vi "GetWheaterData.vi"(11 "Locaion":string="newyork") -> (3 "WeatherString":string)   [LabVIEW 2015]
uses:
  TypeDefs/OpenWeatherMapAPI.Responce.ctl
  <vilib>/httpClient/LabVIEWHTTPClient.lvlib
panel:
  out "error out":errorcluster
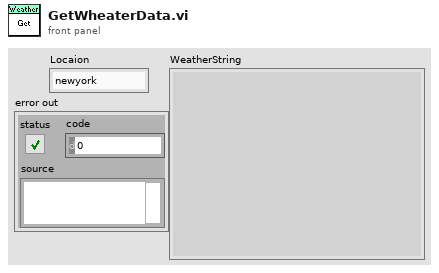
[diagram p1: front panel]
types:
  T1 = typedef "OpenWeatherMapAPI.Responce.ctl" = cluster{"weather":cluster{"main":string, "description":string}[], "main":cluster{"temp":dbl, "pressure":i32, "humidity":i32}, "wind":cluster{"speed":sgl}, "clouds":cluster{"all":i32}, "dt":u64, "sys":cluster{"country":string, "sunrise":u64, "sunset":u64}, "id":i32, "name":string, "cod":i32}
  T2 = cluster{"weather[0]":cluster{"main":string, "description":string}}
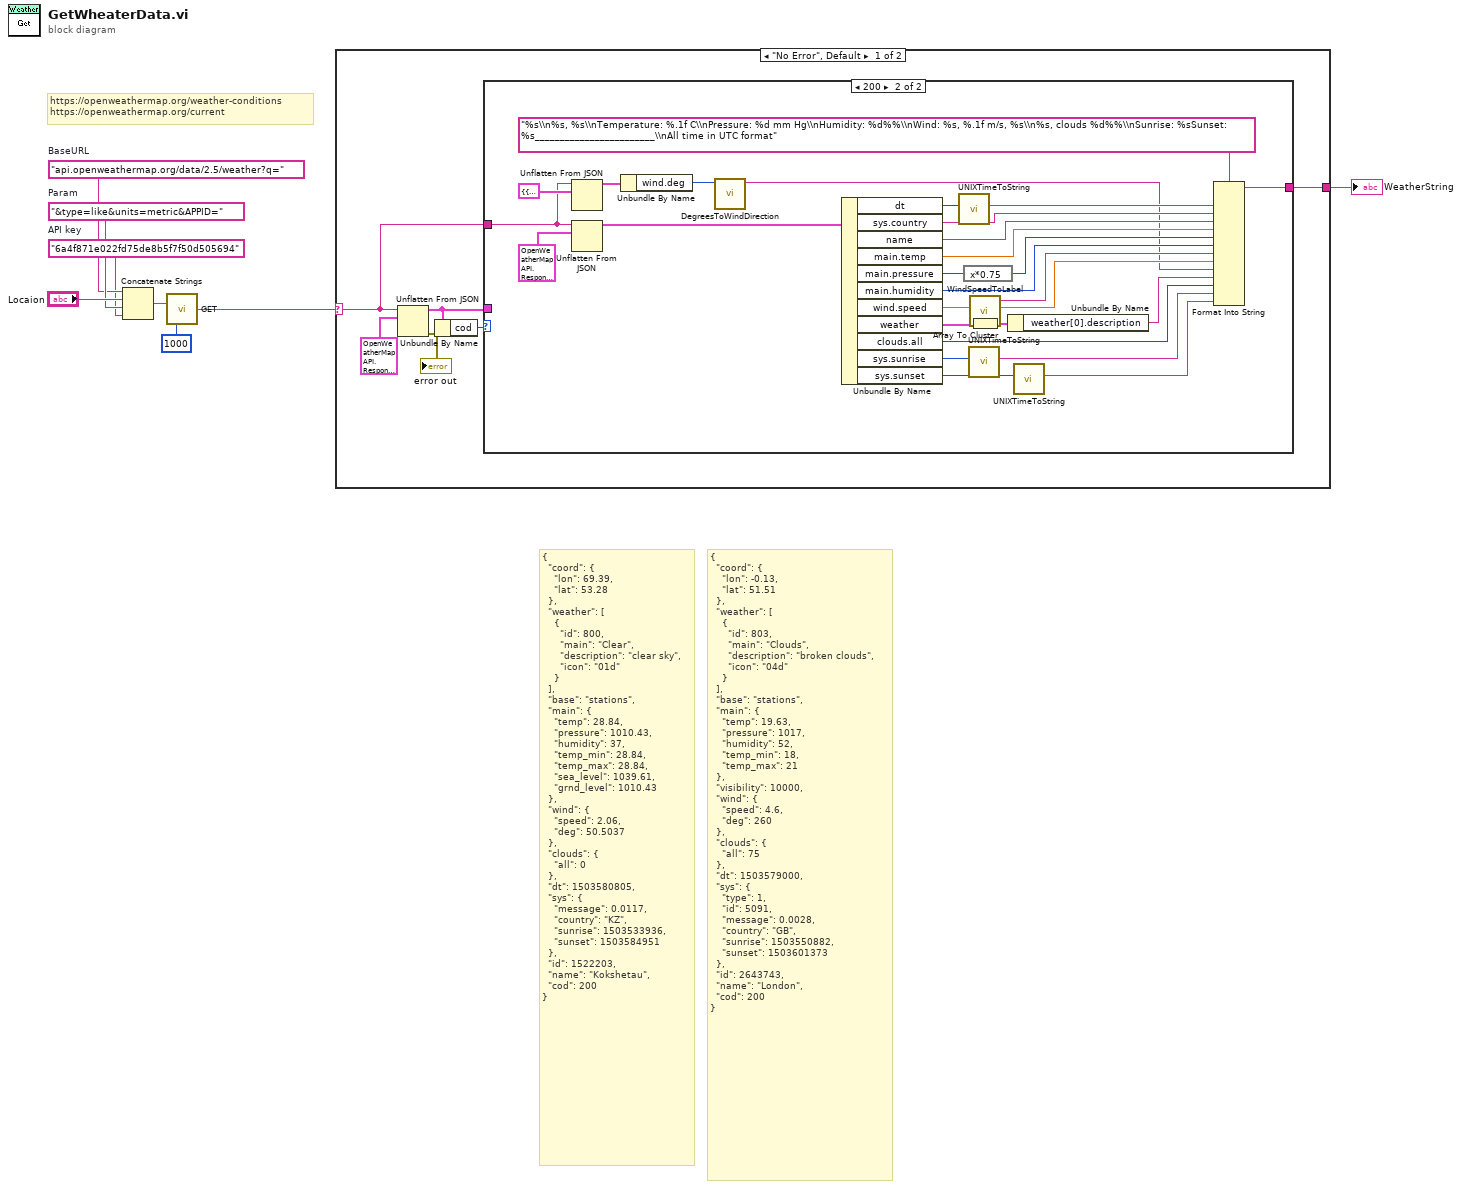
[diagram p0: block diagram]
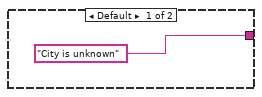
[diagram p2: hidden frame]
diagram:
  w3 = "6a4f871e022fd75de8b5f7f50d505694"  # API key
  w5 = "api.openweathermap.org/data/2.5/weather?q="  # BaseURL
  w6 = "&type=like&units=metric&APPID="  # Param
  # "https://openweathermap.org/weather-conditions\nhttps://openweathermap.org/current"
  # "{\n  \"coord\": {\n    \"lon\": -0.13,\n    \"lat\": 51.51\n  },\n  \"weather\": [\n    {\n      \"id\": 803,\n      \"main\": \"Clouds\",\n      \"description\": \"broken clouds\",\n      \"icon\": \"04d\"\n    }\n  ],\n  \"base\": \"stations\",\n  \"main\": {\n    \"temp\": 19.63,\n    \"pressure\": 1017,\n    \"humidity\": 52,\n    \"temp_min\": 18,\n    \"temp_max\": 21\n  },\n  \"visibility\": 10000,\n  \"wind\": {\n    \"speed\": 4.6,\n    \"deg\": 260\n  },\n  \"clouds\": {\n    \"all\": 75\n  },\n  \"dt\": 1503579000,\n  \"sys\": {\n    \"type\": 1,\n    \"id\": 5091,\n    \"message\": 0.0028,\n    \"country\": \"GB\",\n    \"sunrise\": 1503550882,\n    \"sunset\": 1503601373\n  },\n  \"id\": 2643743,\n  \"name\": \"London\",\n  \"cod\": 200\n}"
  # "{\n  \"coord\": {\n    \"lon\": 69.39,\n    \"lat\": 53.28\n  },\n  \"weather\": [\n    {\n      \"id\": 800,\n      \"main\": \"Clear\",\n      \"description\": \"clear sky\",\n      \"icon\": \"01d\"\n    }\n  ],\n  \"base\": \"stations\",\n  \"main\": {\n    \"temp\": 28.84,\n    \"pressure\": 1010.43,\n    \"humidity\": 37,\n    \"temp_min\": 28.84,\n    \"temp_max\": 28.84,\n    \"sea_level\": 1039.61,\n    \"grnd_level\": 1010.43\n  },\n  \"wind\": {\n    \"speed\": 2.06,\n    \"deg\": 50.5037\n  },\n  \"clouds\": {\n    \"all\": 0\n  },\n  \"dt\": 1503580805,\n  \"sys\": {\n    \"message\": 0.0117,\n    \"country\": \"KZ\",\n    \"sunrise\": 1503533936,\n    \"sunset\": 1503584951\n  },\n  \"id\": 1522203,\n  \"name\": \"Kokshetau\",\n  \"cod\": 200\n}"
  n1 = Concatenate Strings(w5, "Locaion", w6, w3) -> (w7:string)
  n2 = call <vilib>:"GET.vi"("url"=w7, "timeout (10000)"=1000) -> ("body"=w2:string)  [unwired: 10 in, 3 out]
  n3 = case shown="\"No Error\", Default" w2 {
    selector: w2 -> [w11 _]
    tunnel: [w10 _] -> w1
    frame "No Error", Default {
      n4 = Unflatten From JSON(JSON string=w11, type and defaults=T1 {"weather"=[], "main"={"temp"=0.0, "pressure"=0, "humidity"=0}, "wind"={"speed"=0.0}, "clouds"={"all"=0}, "dt"=0, "sys"={"country"="", "sunrise"=0, "sunset"=0}, "id"=0, "name"="", "cod"=0}) -> (value=w13:T1, error out=→"error out":errorcluster)  [unwired: 5 in]
      n5 = Unbundle By Name(w13) -> ("cod"=w14:i32)
      n6 = case shown="200" w14 {
        tunnel: w13 -> [_ _]
        tunnel: ["City is unknown" w16] -> w10
        tunnel: w11 -> [_ w18]
        frame Default {
        }
        frame 200 {
          n7 = Unflatten From JSON(JSON string=w18, type and defaults=cluster{"wind":cluster{"deg":i32}, "cod":i32} {"wind"={"deg"=0}, "cod"=0}) -> (value=w41:cluster{"wind":cluster{"deg":i32}, "cod":i32})  [unwired: 5 in, 1 out]
          n8 = Unflatten From JSON(JSON string=w18, type and defaults=T1 {"weather"=[], "main"={"temp"=0.0, "pressure"=0, "humidity"=0}, "wind"={"speed"=0.0}, "clouds"={"all"=0}, "dt"=0, "sys"={"country"="", "sunrise"=0, "sunset"=0}, "id"=0, "name"="", "cod"=0}) -> (value=w38:T1)  [unwired: 5 in, 1 out]
          n9 = Unbundle By Name(w41) -> ("wind.deg"=w40:i32)
          n10 = call "DegreesToWindDirection.vi"("Degrees"=w40) -> ("WindDirection"=w17:string)  [unwired: 10 in]
          n11 = Unbundle By Name(w38) -> ("dt"=w37:u64, "sys.country"=w34:string, "name"=w33:string, "main.temp"=w32:dbl, "main.pressure"=w31:i32, "main.humidity"=w29:i32, "wind.speed"=w27:sgl, "weather"=w26:cluster{"main":string, "description":string}[], "clouds.all"=w23:i32, "sys.sunrise"=w22:u64, "sys.sunset"=w20:u64)
          n12 = call "UNIXTimeToString.vi"("dt"=w37) -> ("DateTime"=w36:string)  [unwired: 10 in]
          n13 = expression code="x*0.75"(w31) -> (w30:i32)
          n14 = call "UNIXTimeToString.vi"("dt"=w22) -> ("DateTime"=w21:string)  [unwired: 10 in]
          n15 = call "WindSpeedToLabel.vi"("Wind speed (m/sec)"=w27) -> ("Label"=w28:string)  [unwired: 10 in]
          n16 = Array To Cluster(array=w26) -> (cluster=w25:T2)
          n17 = Unbundle By Name(w25) -> ("weather[0].description"=w24:string)
          n18 = call "UNIXTimeToString.vi"("dt"=w20) -> ("DateTime"=w19:string)  [unwired: 10 in]
          n19 = Format Into String(format string="%s\\n%s, %s\\nTemperature: %.1f C\\nPressure: %d mm Hg\\nHumidity: %d%%\\nWind: %s, %.1f m/s, %s\\n%s, clouds %d%%\\nSunrise: %sSunset: %s________________________\\nAll time in UTC format", w36, w34, w33, w32, w30, w29, w28, w27, w17, w24, w23, w21, w19) -> (resulting string=w16:string)  [unwired: 2 in, 1 out]
        }
      }
    }
    frame "{}" {
    }
  }
  "WeatherString" <- w1
